vi "Lift.vi"(0 "left encoder":dbl, 1 "right encoder":dbl, 3 "move to":bool, 4 "move to distance":dbl, 5 "reset max":bool, 7 "last max difference":dbl, 8 "left output range":cluster{"output high":dbl, "output low":dbl}={"output high"=100.0, "output low"=-100.0} {"output low" format="%.2f"; "output high" format="%.2f"}, 9 "left PID gains":T1={"proportional gain (Kc)"=1.0, "integral time (Ti, min)"=0.01, "derivative time (Td, min)"=0.0} {"derivative time (Td, min)" format="%.3f"; "integral time (Ti, min)" format="%.3f"; "proportional gain (Kc)" format="%.3f"}, 10 "constant":dbl, 12 "right output range":cluster{"output high":dbl, "output low":dbl}={"output high"=100.0, "output low"=-100.0} {"output low" format="%.2f"; "output high" format="%.2f"}, 13 "right PID gains":T1={"proportional gain (Kc)"=1.0, "integral time (Ti, min)"=0.01, "derivative time (Td, min)"=0.0} {"derivative time (Td, min)" format="%.3f"; "integral time (Ti, min)" format="%.3f"; "proportional gain (Kc)" format="%.3f"}) -> (14 "lift motor left":dbl=-0.25, 15 "encoder count left":dbl, 16 "lift motor right":dbl=0.5, 17 "encoder count right":dbl, 23 "left to target difference":dbl, 27 "max difference":dbl)   [LabVIEW 2014]
uses:
  <vilib>/addons/control/pid/pid.llb/PID (DBL).vi
  <vilib>/addons/control/pid/NI_PID_pid.lvlib
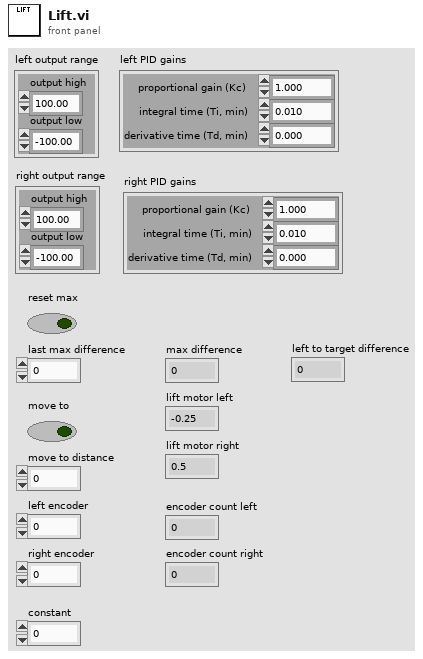
[diagram p1: front panel]
types:
  T1 = cluster{"proportional gain (Kc)":dbl, "integral time (Ti, min)":dbl, "derivative time (Td, min)":dbl}
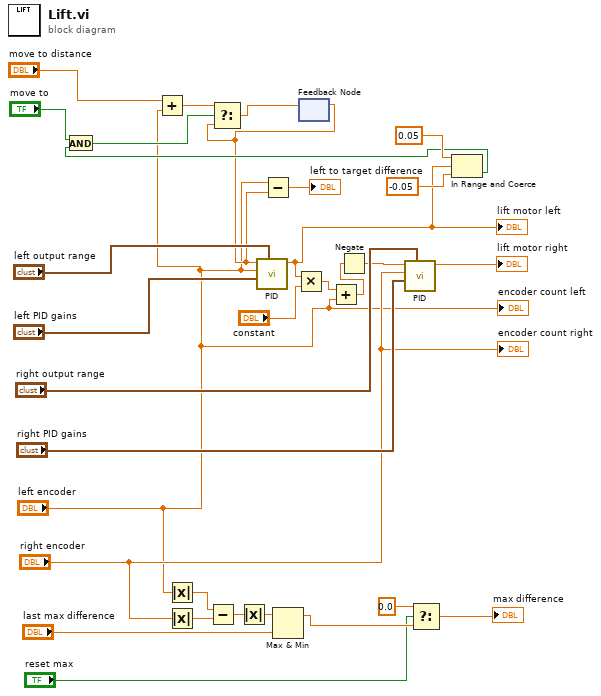
[diagram p0: block diagram]
diagram:
  n1 = Add(x="move to distance", y="left encoder") -> (x+y=w12:dbl)
  n2 = Absolute Value(x="left encoder") -> (abs(x)=w24:dbl)
  n3 = Absolute Value(x="right encoder") -> (abs(x)=w23:dbl)
  n4 = Subtract(x=w24, y=w23) -> (x-y=w21:dbl)
  n5 = Absolute Value(x=w21) -> (abs(x)=w20:dbl)
  n6 = Max & Min(x=w20, y="last max difference") -> (max(x,y)=w19:dbl)  [unwired: 1 out]
  n7 = feedback #1() -> (w6:dbl)  [unwired: 1 in]
  n8 = call-poly <vilib>:"PID.vi"("output range"="left output range", "PID gains"="left PID gains", "process variable"="left encoder", "setpoint"=w6) -> ("output"=w5:dbl)  [unwired: 6 in, 1 out]
  "lift motor left" <- w5
  n9 = Subtract(x="left encoder", y=w6) -> (x-y=→"left to target difference":dbl)
  n10 = Multiply(x=w5, y="constant") -> (x*y=w1:dbl)
  n11 = Add(x=w1, y="left encoder") -> (x+y=w3:dbl)
  n12 = Negate(x=w3) -> (-x=w26:dbl)
  n13 = call-poly <vilib>:"PID.vi"("output range"="right output range", "PID gains"="right PID gains", "process variable"="right encoder", "setpoint"=w26) -> ("output"=→"lift motor right":dbl)  [unwired: 6 in, 1 out]
  n14 = Select(t=0.0, s="reset max", f=w19) -> (s? t:f=→"max difference":dbl)
  n15 = In Range and Coerce(upper limit=0.05, x=w5, lower limit=-0.05) -> (In Range?=w13:bool)  [unwired: 1 out]
  n16 = And(x="move to", y=w13) -> (x .and. y?=w10:bool)
  n17 = Select(t=w12, s=w10, f=w6) -> (s? t:f=w11:dbl)
  n18 = feedback-in #1(w11) -> ()
  "encoder count left" <- "left encoder"
  "encoder count right" <- "right encoder"
